vi "Change in Product Installers.vi"(8 "error in (no error)":errorcluster, 10 "Product Installers":cluster{"Key":string, "Version":string}[](array[cluster]), 11 "Bundle Builder in":refnum<class "Bundle Builder.lvclass">) -> (0 "error out":errorcluster, 1 "Custom Actions File Names":string[](array[string]), 2 "Product List File Names":string[](array[string]), 3 "Bundle Builder out":refnum<class "Bundle Builder.lvclass">, 4 "Bundle Filename":string)   [LabVIEW 2020, in "Bundle Builder.lvclass"]
uses:
  Bundle Builder.lvclass
  Bundle Builder.lvclass/Bundle Builder.ctl
  4f63f28f-5265-4602-8317-7e5f909f2807.vi
  5d65ce95-3f27-4ad9-b4d3-753b2ea8e44f.vi
  <vilib>/Comparison/Equal/Equal Functor/Equal Functor.lvclass
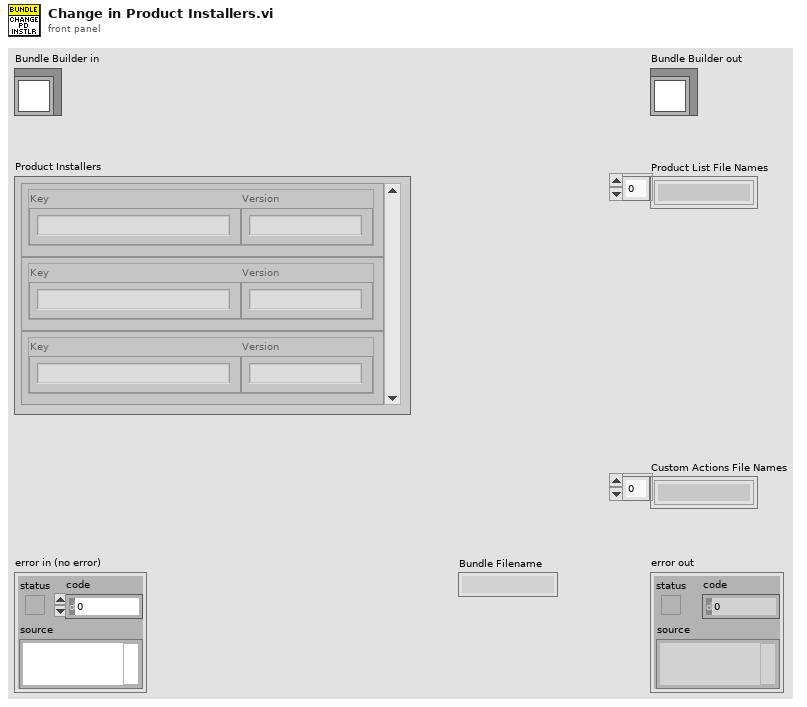
[diagram p1: front panel]
types:
  T1 = enum16{"All Elements Deleted", "Element Deleted", "Element Inserted", "Element Content Changed"}
  T2 = cluster{"Display Name":string, "Type":enum16{"NI Installer", "Custom Installer"}, "Install Commands":cluster{"Path":string, "Parameters":string, "Successful Exit Codes":string, "Log Command":cluster{"Flag":string, "File Name":string}}[], "Uninstall Commands":cluster{"Path":string, "Parameters":string, "Successful Exit Codes":string, "Log Command":cluster{"Flag":string, "File Name":string}}[]}[]
  T3 = cluster{"Display Name":string, "Type":enum16{"NI Installer", "Custom Installer"}, "Install Commands":cluster{"Path":string, "Parameters":string, "Successful Exit Codes":string, "Log Command":cluster{"Flag":string, "File Name":string}}[], "Uninstall Commands":cluster{"Path":string, "Parameters":string, "Successful Exit Codes":string, "Log Command":cluster{"Flag":string, "File Name":string}}[]}
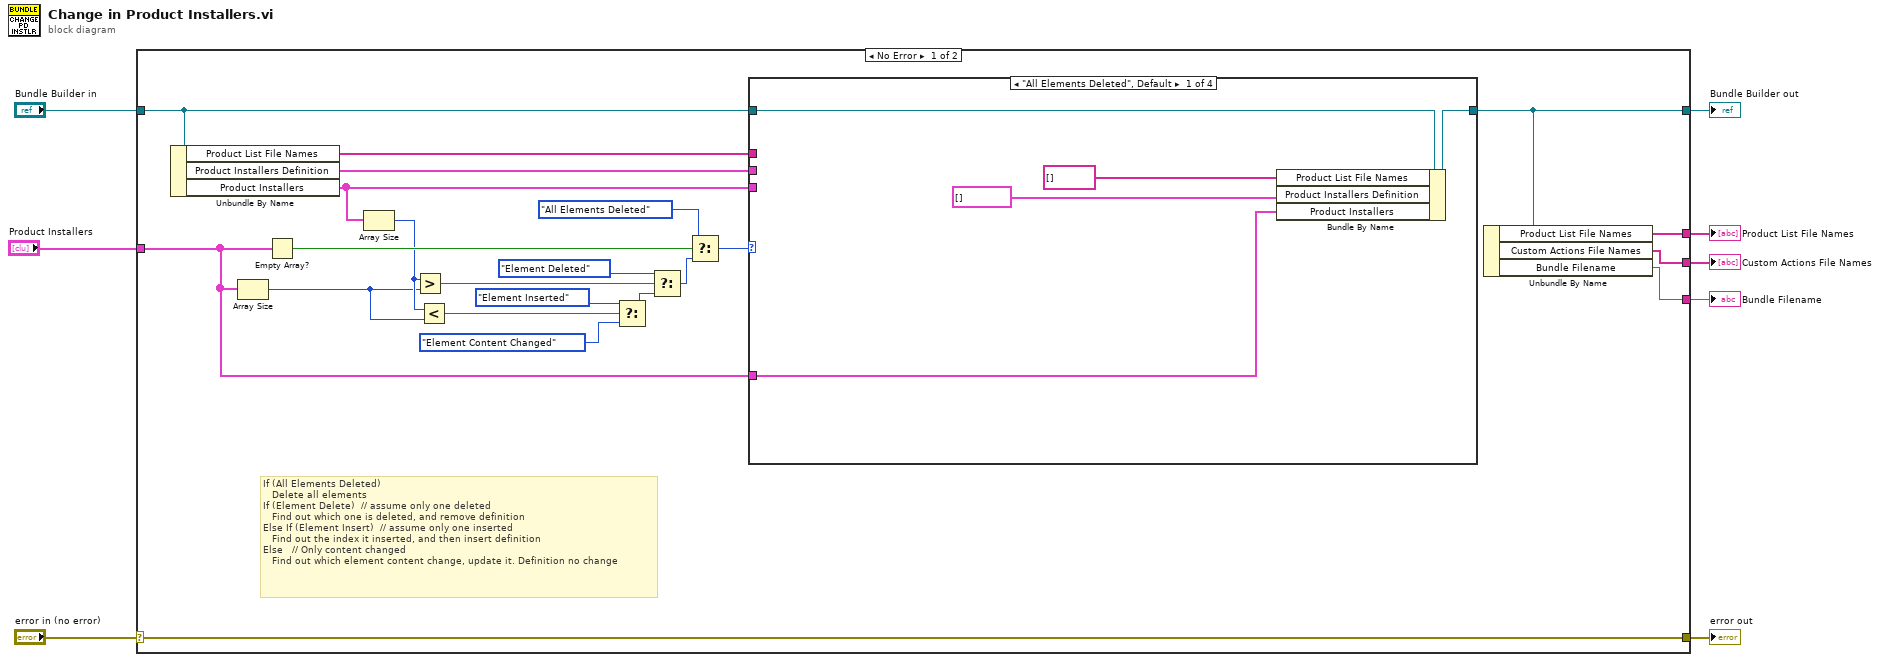
[diagram p0: block diagram]
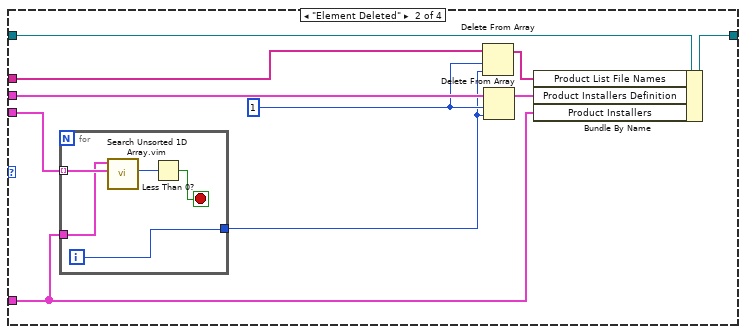
[diagram p2: hidden frame]
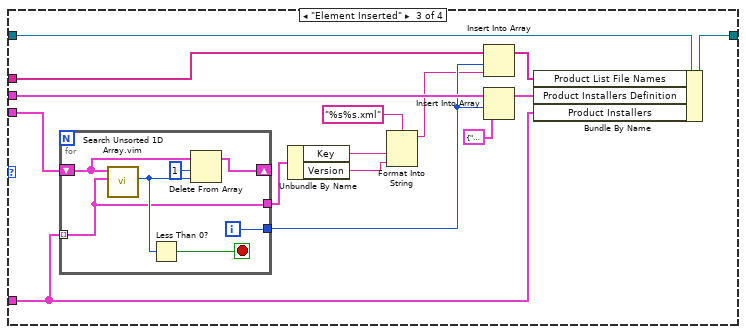
[diagram p3: hidden frame]
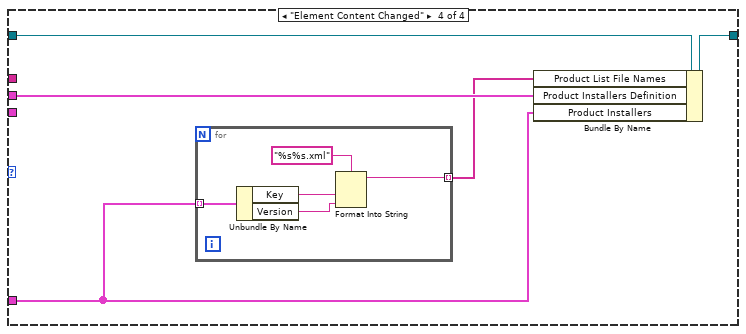
[diagram p4: hidden frame]
diagram:
  n1 = case shown="No Error" "error in (no error)" {
    selector: "error in (no error)" -> [w30 w84]
    tunnel: [w30 w84] -> w7
    tunnel: [w13 w83] -> w5
    tunnel: "Bundle Builder in" -> [w17 w83]
    tunnel: "Product Installers" -> [w16 _]
    tunnel: [w11 _] -> w3
    tunnel: [w10 _] -> w2
    tunnel: [w9 _] -> w1
    frame No Error {
      # "If (All Elements Deleted)\n   Delete all elements\nIf (Element Delete)  // assume only one deleted\n   Find out which one is deleted, and remove definition\nElse If (Element Insert)  // assume only one inserted\n   Find out the index it inserted, and then insert definition\nElse   // Only content changed\n   Find out which element content change, update it. Definition no change"
      n2 = Unbundle By Name(w17) -> ("Product List File Names"=w12:string[], "Product Installers Definition"=w14:T2, "Product Installers"=w15:cluster{"Key":string, "Version":string}[])
      n3 = Array Size(array=w16) -> (size(s)=w23:i32)
      n4 = Empty Array?(array=w16) -> (empty?=w29:bool)
      n5 = Array Size(array=w15) -> (size(s)=w24:i32)
      n6 = Greater?(x=w24, y=w23) -> (0:w25:bool)
      n7 = Less?(x=w24, y=w23) -> (x < y?=w20:bool)
      n8 = Select(t=T1."Element Inserted", s=w20, f=T1."Element Content Changed") -> (s? t:f=w22:T1)
      n9 = Select(t=T1."Element Deleted", s=w25, f=w22) -> (s? t:f=w26:T1)
      n10 = Select(t=T1."All Elements Deleted", s=w29, f=w26) -> (s? t:f=w18:T1)
      n11 = case shown="\"All Elements Deleted\", Default" w18 {
        tunnel: w17 -> [w35 w45 w65 w77]
        tunnel: [w34 w44 w64 w76] -> w13
        tunnel: w16 -> [w32 w40 w59 w74]
        tunnel: w15 -> [_ w43 w63 _]
        tunnel: w14 -> [_ w42 w62 w75]
        tunnel: w12 -> [_ w39 w58 _]
        frame "All Elements Deleted", Default {
          n12 = Bundle By Name(cluster=w35, "Product List File Names"=string[] [], "Product Installers Definition"=T2 [], "Product Installers"=w32) -> (w34:refnum<class "Bundle Builder.lvclass">)
        }
        frame "Element Deleted" {
          w37 = 1 ("length")
          n13 = for {
            tunnel: w43 -> [w50] mode=indexing
            tunnel: w40 -> [w49]
            tunnel: [w46] -> w36
            i -> [w46]
            stop <- w48 stop-if-true
            n14 = call "Search Unsorted 1D Array.vim"("element"=w50, "unsorted 1D array"=w49) -> ("index of element"=w47:i32)  [unwired: 9 in]
            n15 = Less Than 0?(x=w47) -> (x < 0?=w48:bool)
          }
          n16 = Delete From Array(array=w39, length=w37, index=w36) -> (array with subset deleted=w38:string[])  [unwired: 1 out]
          n17 = Delete From Array(array=w42, length=w37, index=w36) -> (array with subset deleted=w41:T2)  [unwired: 1 out]
          n18 = Bundle By Name(cluster=w45, "Product List File Names"=w38, "Product Installers Definition"=w41, "Product Installers"=w40) -> (w44:refnum<class "Bundle Builder.lvclass">)
        }
        frame "Element Inserted" {
          n19 = for {
            tunnel: w59 -> [w66] mode=indexing
            tunnel: [w71] -> w57
            shift-right: [w67] -> _
            shift-left: w63 -> [w70]
            tunnel: [w66] -> w56
            i -> [w71]
            stop <- w72 stop-if-true
            n20 = call "Search Unsorted 1D Array.vim"("element"=w66, "unsorted 1D array"=w70) -> ("index of element"=w69:i32)  [unwired: 9 in]
            n21 = Less Than 0?(x=w69) -> (x < 0?=w72:bool)
            n22 = Delete From Array(array=w70, length=1, index=w69) -> (array with subset deleted=w67:cluster{"Key":string, "Version":string}[])  [unwired: 1 out]
          }
          n23 = Unbundle By Name(w56) -> ("Key"=w54:string, "Version"=w53:string)
          n24 = Format Into String(format string="%s%s.xml", w54, w53) -> (resulting string=w52:string)  [unwired: 2 in, 1 out]
          n25 = Insert Into Array(array=w58, index=w57, new element=w52) -> (w51:string[])
          n26 = Insert Into Array(array=w62, index=w57, new element=T3 {"Display Name"="", "Type"=enum."NI Installer", "Install Commands"=[], "Uninstall Commands"=[]} ("new element/subarray")) -> (w61:T2)
          n27 = Bundle By Name(cluster=w65, "Product List File Names"=w51, "Product Installers Definition"=w61, "Product Installers"=w59) -> (w64:refnum<class "Bundle Builder.lvclass">)
        }
        frame "Element Content Changed" {
          n28 = for {
            tunnel: w74 -> [w79] mode=indexing
            tunnel: [w78] -> w73 mode=indexing
            n29 = Unbundle By Name(w79) -> ("Key"=w81:string, "Version"=w80:string)
            n30 = Format Into String(format string="%s%s.xml", w81, w80) -> (resulting string=w78:string)  [unwired: 2 in, 1 out]
          }
          n31 = Bundle By Name(cluster=w77, "Product List File Names"=w73, "Product Installers Definition"=w75, "Product Installers"=w74) -> (w76:refnum<class "Bundle Builder.lvclass">)
        }
      }
      n32 = Unbundle By Name(w13) -> ("Product List File Names"=w11:string[], "Custom Actions File Names"=w10:string[], "Bundle Filename"=w9:string)
    }
    frame Error {
    }
  }
  "error out" <- w7
  "Bundle Builder out" <- w5
  "Product List File Names" <- w3
  "Custom Actions File Names" <- w2
  "Bundle Filename" <- w1
